vi "main.vi"() -> ()   [LabVIEW 2020]
doc: "Take photo if matching template."
uses:
  <vilib>/userDefined/High Color/IMAQdx.ctl
  <vilib>/Utility/error.llb/DialogType.ctl
  controls/Car Wash Data.ctl
  controls/Car Wash Entry Console.ctl
  controls/Car Wash Led.ctl
panel:
  in  "Stop program":bool
  in  "Tab Control":enum32{"Controls", "Statistics", "Admin Panel"}(tab)
  out "Reading ID":bool
  in  "Car ID":string
  in  "Car Position Slider":u16(slide) scale=0.0..4.0
  out "Under Body Wash":bool
  out "Bug Remover":bool
  out "Pre-Soak":bool
  out "High Pressure Wash":bool
  out "Low Pressure Wax":bool
  out "Spot Free Rinse":bool
  out "Tire Shine Foam":bool
  out "Air Dry":bool
  out "Vehicle Out Of Position":bool
  out "Elapsed Time":dbl format="%#_2g"
  out "Wash Entry":bool
  in  "Start":bool
  in  "Entry Console":T1
  out "Cleanest Car ID":string[](array[string])
  out "Histogram":cluster{"Options (1-8)":i32[], "Array":i64[]}(graph)
  out "Database":string[][](table)
  in  "Choose camera":T2="cam2"
  out "Current ID":string
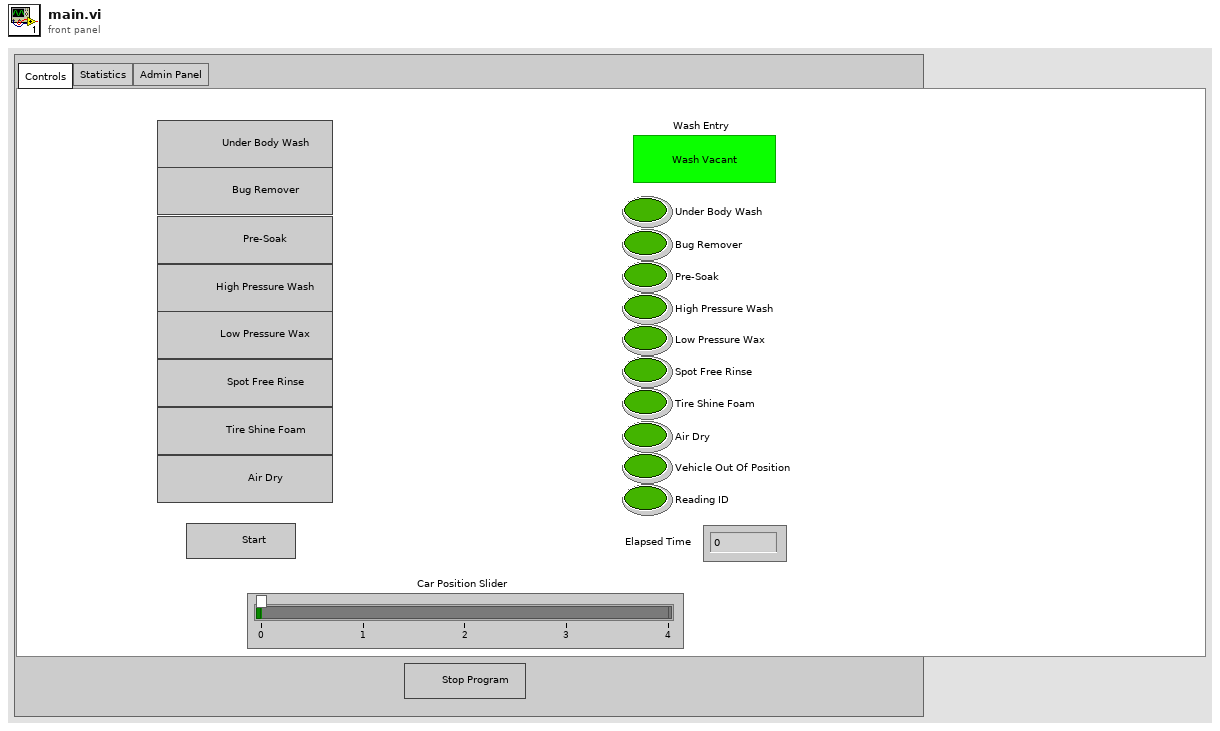
[diagram p1: front panel]
types:
  T1 = cluster{"Under Body Wash Button":bool, "Bug Remover Button":bool, "Pre-Soak Button":bool, "High Pressure Wash Button":bool, "Low Pressure Wax Button":bool, "Spot Free Rinse Button":bool, "Tire Shine Foam Button":bool, "Air Dry Button":bool}
  T2 = typedef "IMAQdx.ctl" = refnum<k21>
  T3 = enum32{"Invalid", "Standard", "Closed", "Hidden", "Minimized", "Maximized"}
  T4 = enum32{"invalid app kind", "Development System", "Run Time System", "Student Edition", "Embedded LabVIEW", "Evaluation", "Custom"}
  T5 = enum8{"Enabled", "Disabled", "Disabled and Grayed Out"}
  T6 = typedef "Car Wash Entry Console.ctl" = cluster{"Under Body Wash Button":bool, "Bug Remover Button":bool, "Pre-Soak Button":bool, "High Pressure Wash Button":bool, "Low Pressure Wax Button":bool, "Spot Free Rinse Button":bool, "Tire Shine Foam Button":bool, "Air Dry":bool}
  T7 = typedef "Car Wash Led.ctl" = cluster{"Under Body Wash":bool, "Bug Remover":bool, "Pre-Soak":bool, "High Pressure Wash":bool, "Low Pressure Wax":bool, "Spot Free Rinse":bool, "Tire Shine Foam":bool, "Air Dry":bool, "Vehicle out If Position":bool, "Wash Entry":bool, "Reading ID":bool}
  T8 = typedef "Car Wash Data.ctl" = cluster{"Entry Console":T6, "Car Wash Display":cluster{"Timer":dbl, "Reset Stoper":bool, "LED":T7, "Elapsed Time":dbl}, "Car Position Slider":u16, "Run Mode":bool}
  T9 = cluster{"Core":cluster{"Current VI Reference":refnum<vi>, "Close Panel on Exit?":bool}, "Car Wash Data":T8, "Car ID":string, "SQLite Connection":refnum<class "Connection.lvclass">}
  T10 = typedef "DialogType.ctl" = u16
  T11 = cluster{"Current VI Reference":refnum<vi>, "Close Panel on Exit?":bool}
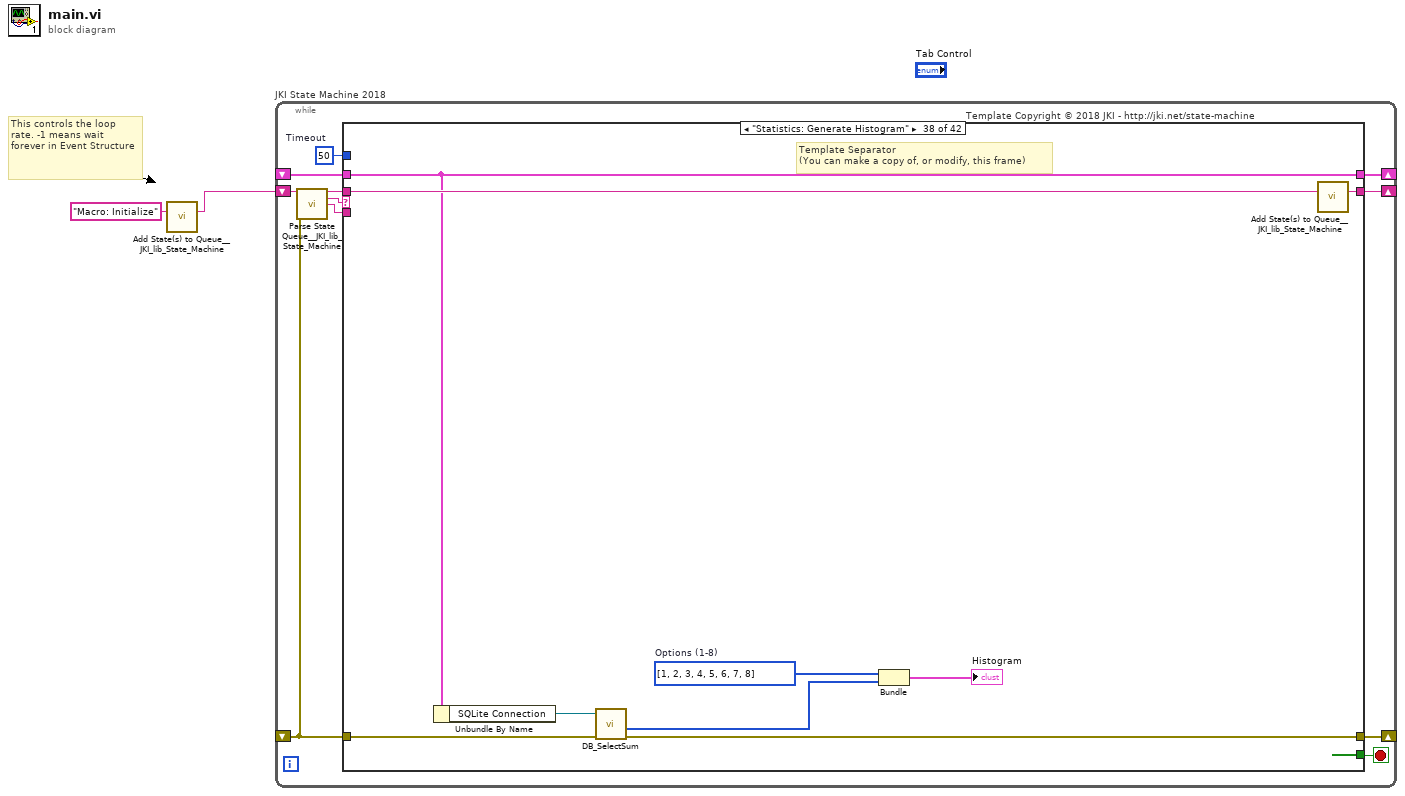
[diagram p0: block diagram]
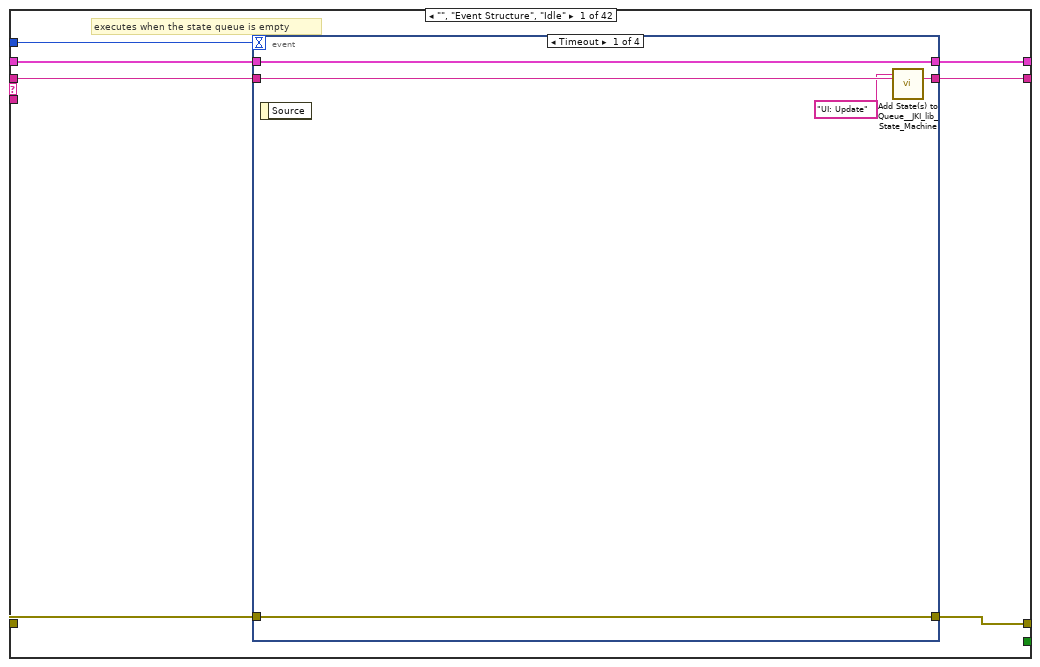
[diagram p2: hidden frame]
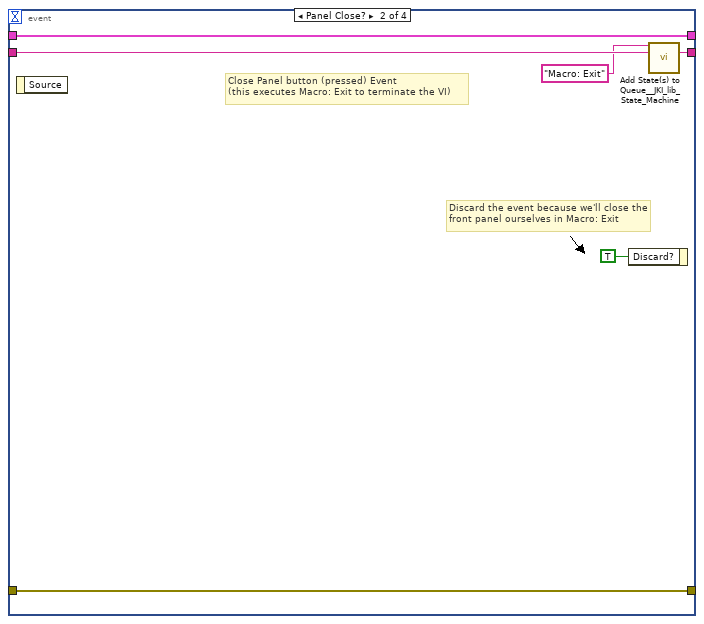
[diagram p3: hidden frame]
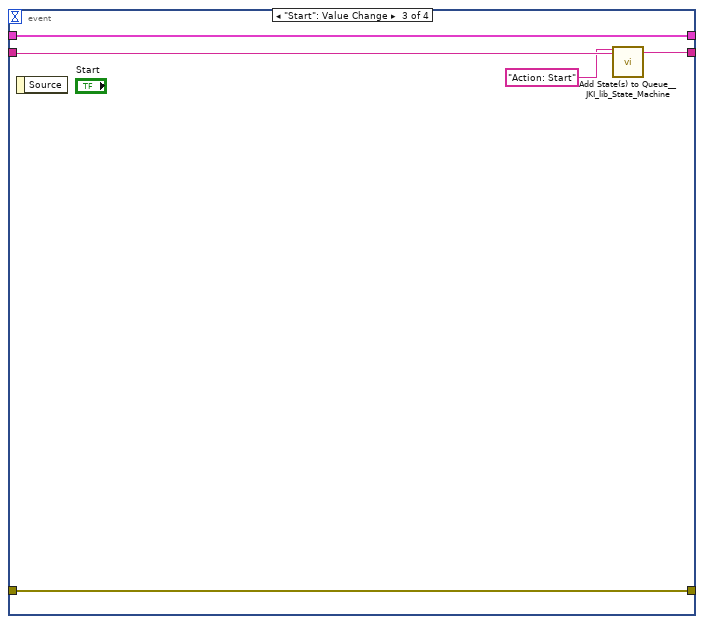
[diagram p4: hidden frame]
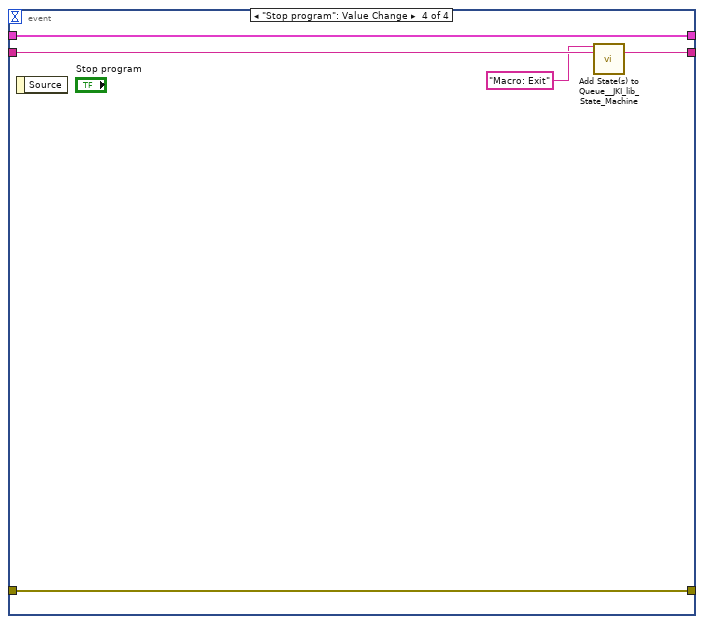
[diagram p5: hidden frame]
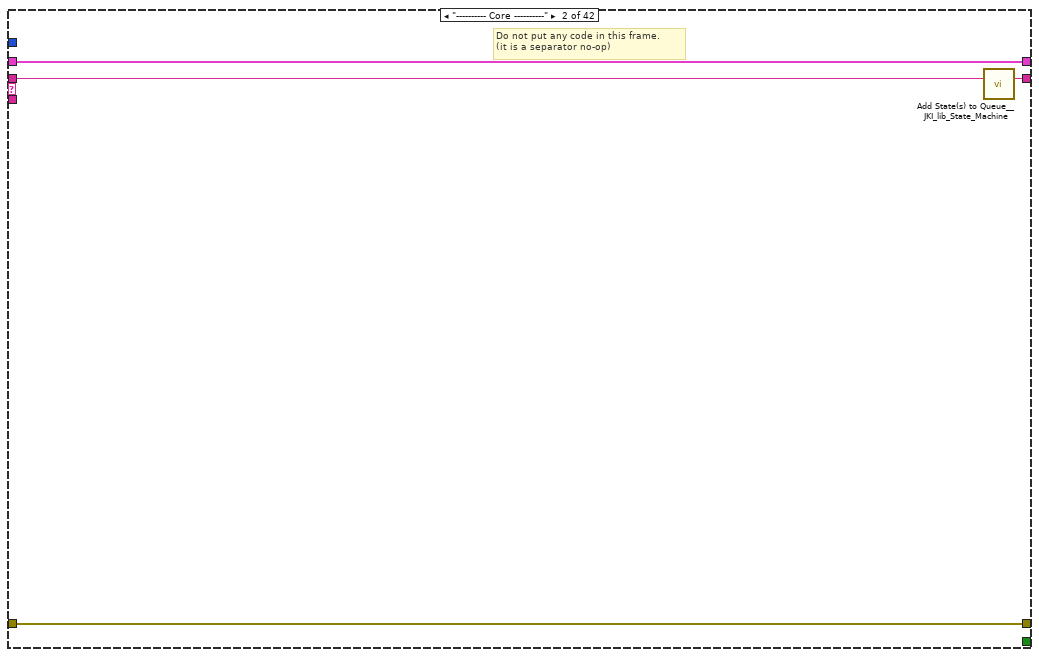
[diagram p6: hidden frame]
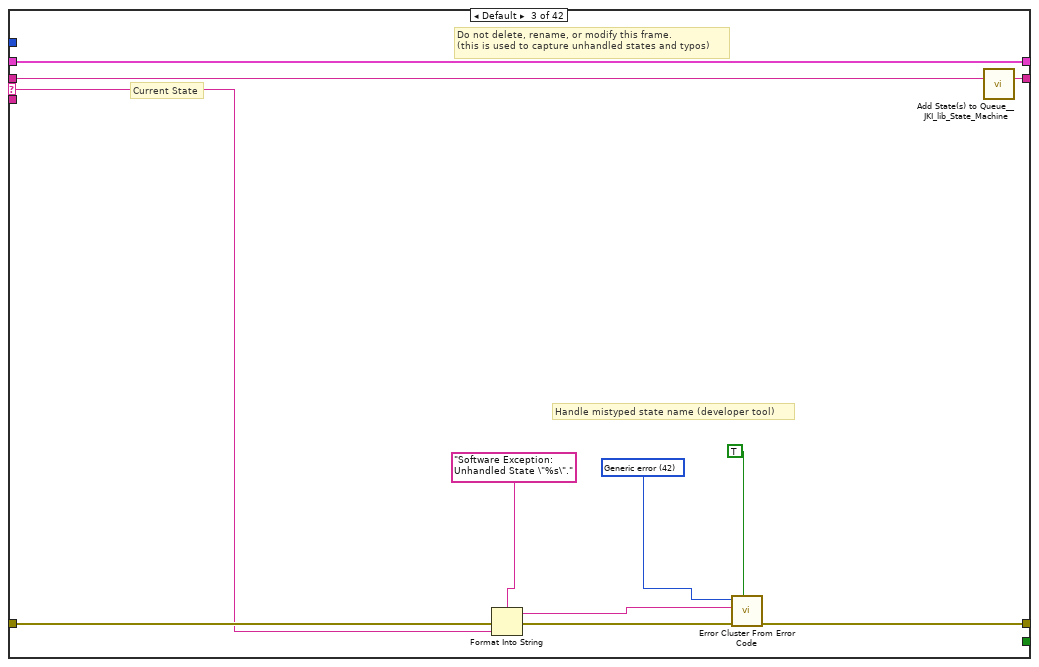
[diagram p7: hidden frame]
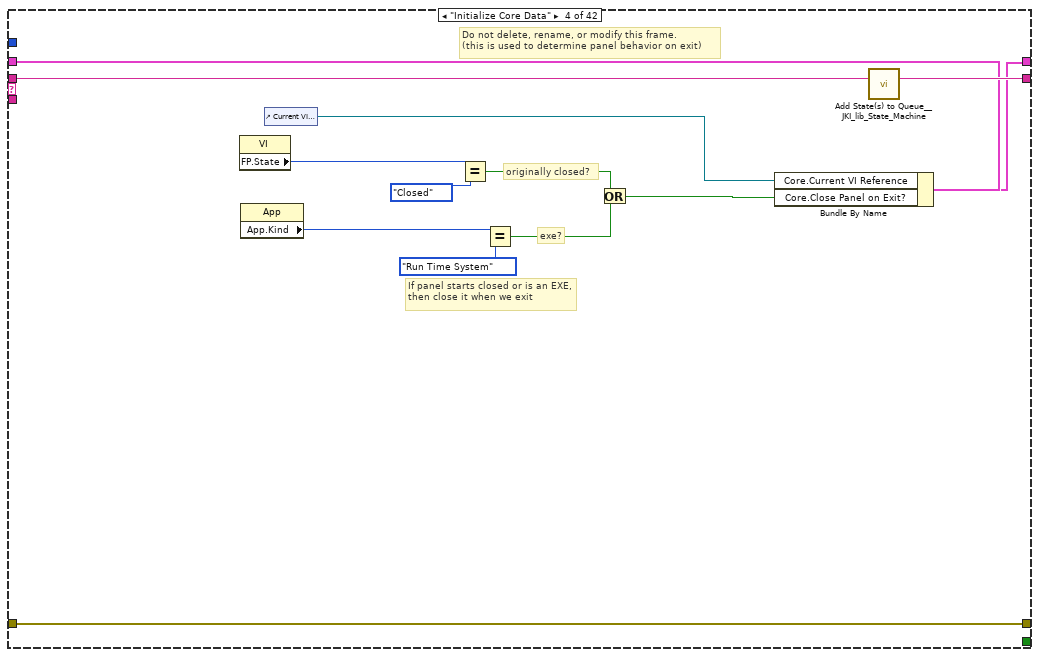
[diagram p8: hidden frame]
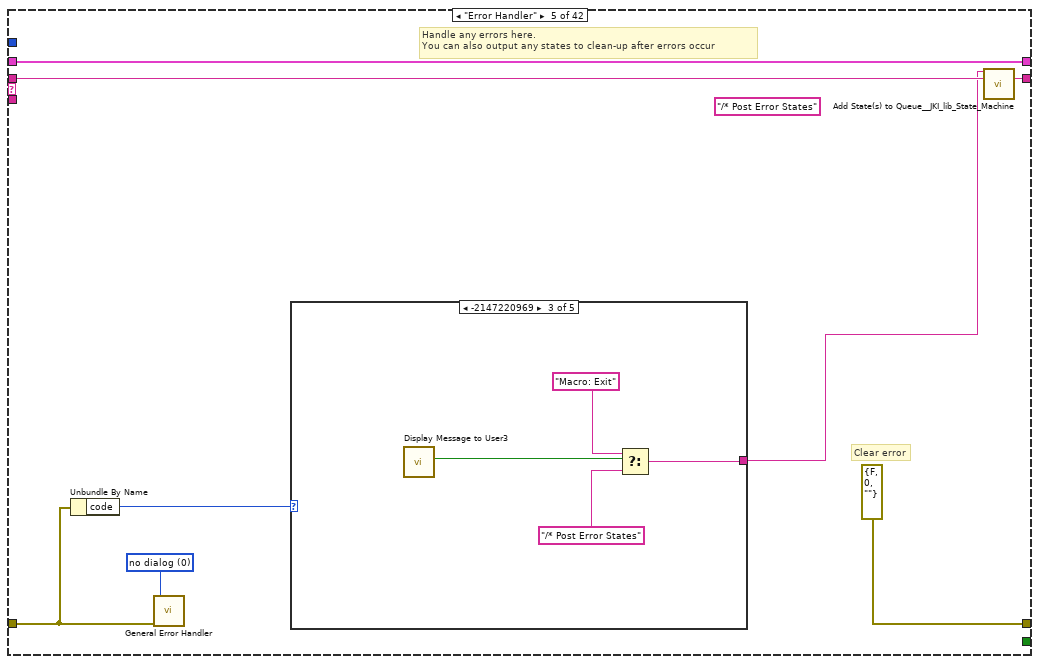
[diagram p9: hidden frame]
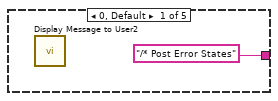
[diagram p10: hidden frame]
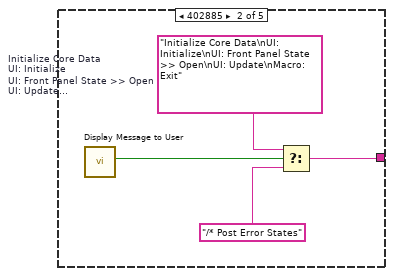
[diagram p11: hidden frame]
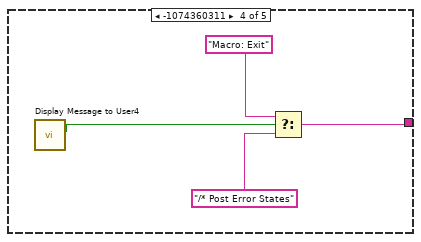
[diagram p12: hidden frame]
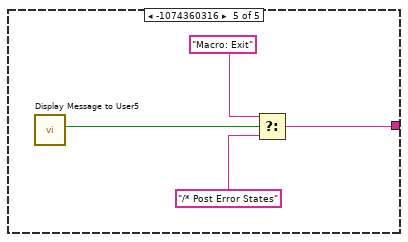
[diagram p13: hidden frame]
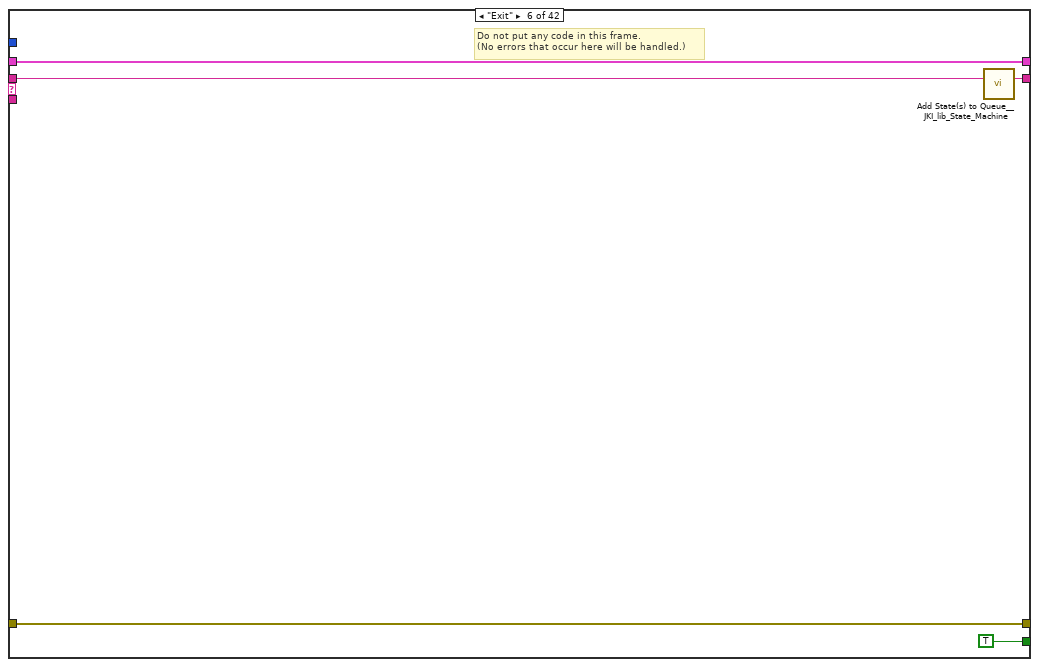
[diagram p14: hidden frame]
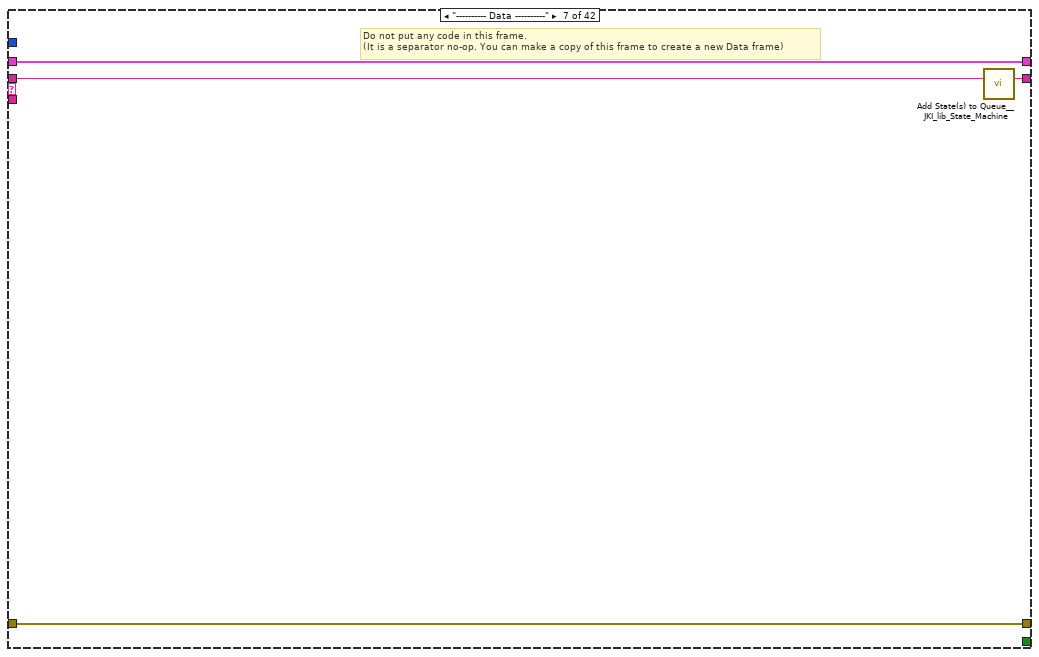
[diagram p15: hidden frame]
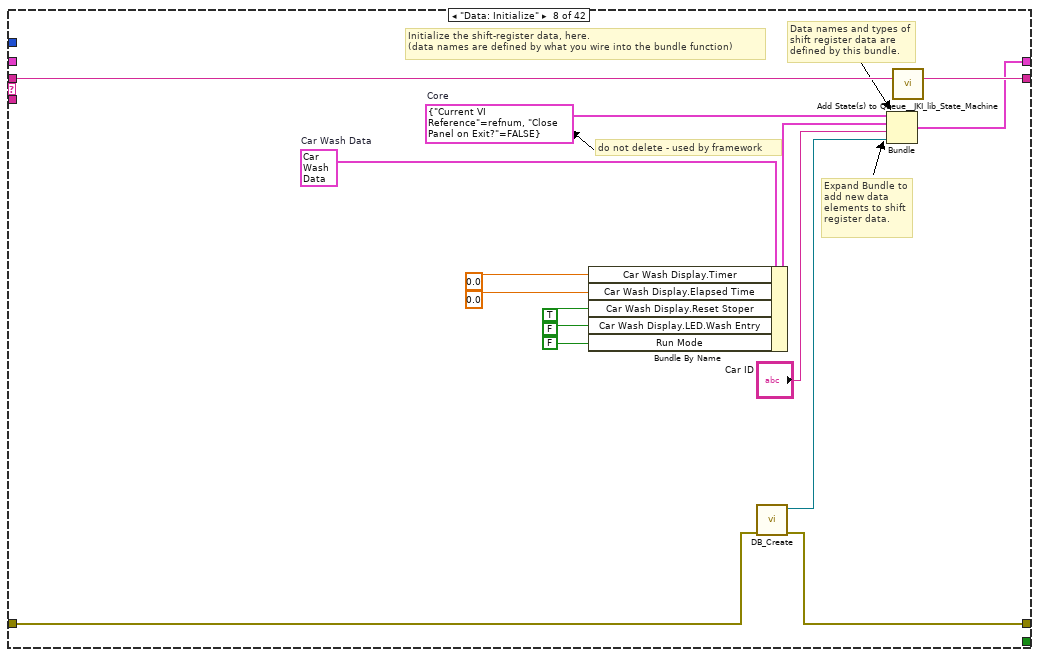
[diagram p16: hidden frame]
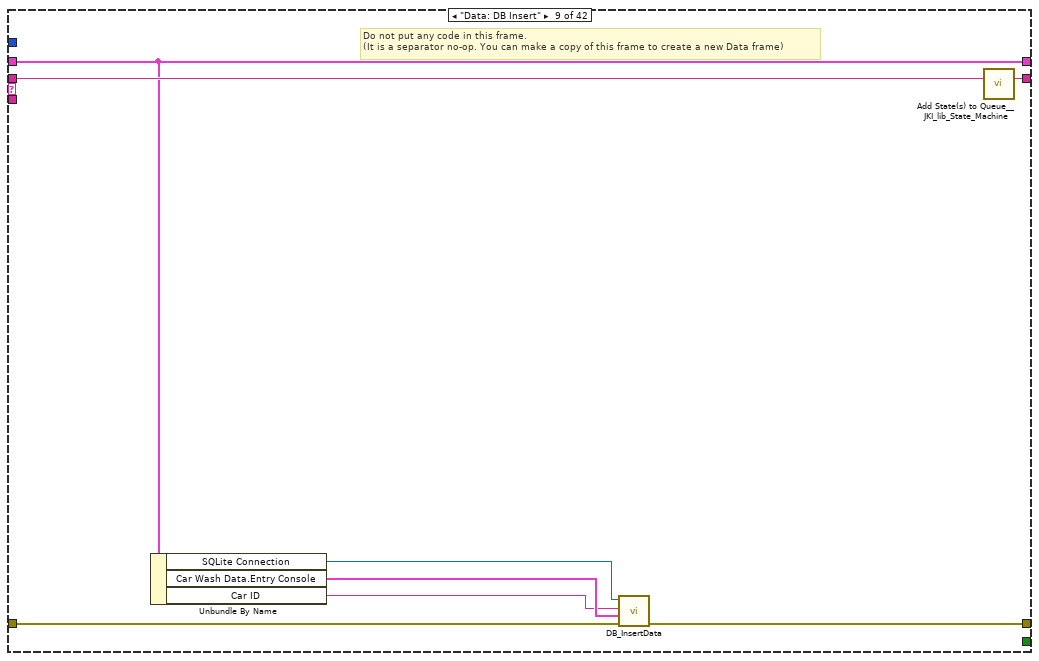
[diagram p17: hidden frame]
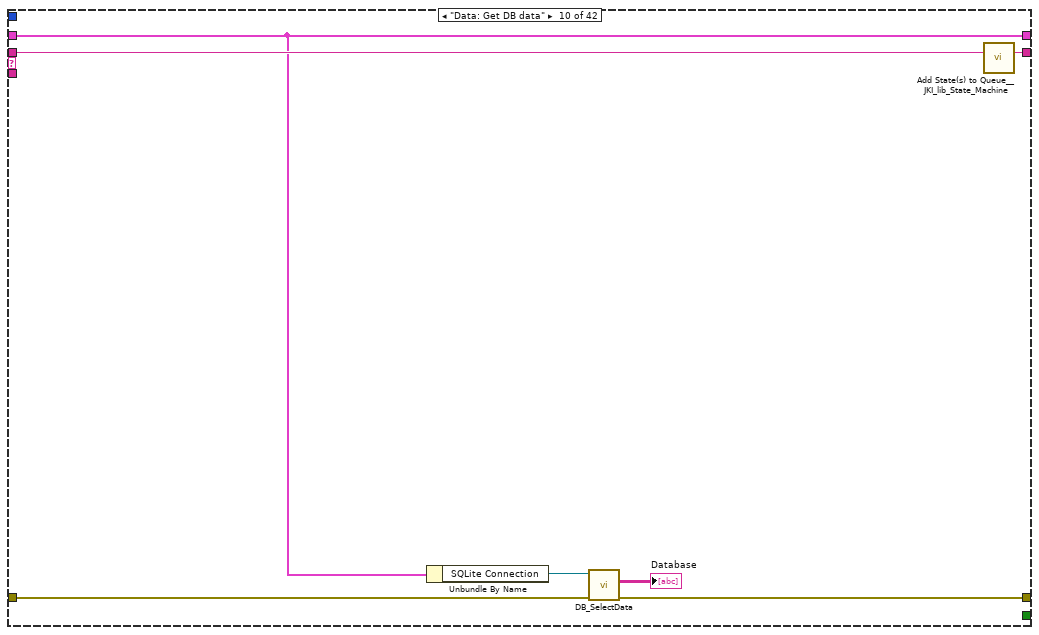
[diagram p18: hidden frame]
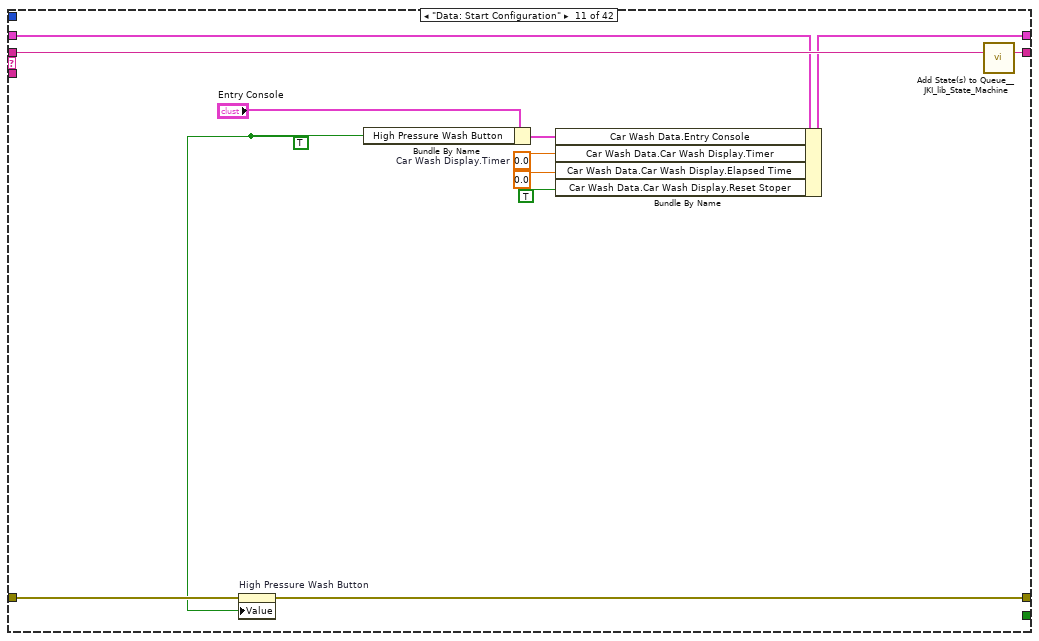
[diagram p19: hidden frame]
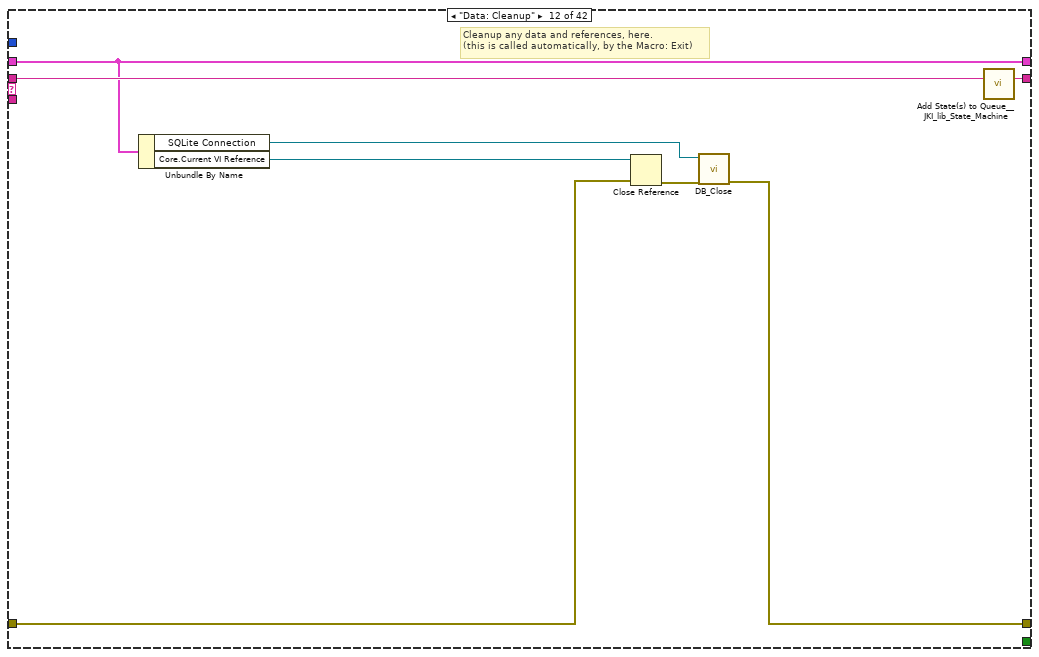
[diagram p20: hidden frame]
diagram:
  # "This controls the loop rate. -1 means wait forever in Event Structure"
  n1 = call <vilib>:"Add State(s) to Queue__JKI_lib_State_Machine.vi"("State(s) in (\"\")"="Macro: Initialize") -> ("States Out"=w2:string)  [unwired: 14 in]
  n2 = while "JKI State Machine 2018" {
    shift-right: [w6] -> _
    shift-left: _ -> [w5]
    shift-right: [w9] -> _
    shift-left: _ -> [w3]
    shift-right: [w8] -> _
    shift-left: w2 -> [w10]
    stop <- w7 stop-if-true
    w4 = 50  # Timeout
    # "Template Copyright © 2018 JKI - http://jki.net/state-machine"
    n3 = call <vilib>:"Parse State Queue__JKI_lib_State_Machine.vi"("State Queue"=w10, "Error In (no error)"=w3) -> ("Remaining States"=w12:string, "Current State"=w13:string, "Arguments"=w11:string)  [unwired: 11 in]
    n4 = case shown="\"Statistics: Generate Histogram\"" w13 {
      selector: w13 -> [_ _ w46 _ _ _ _ _ _ _ _ _ _ _ _ _ _ _ _ _ _ _ _ _ _ _ _ _ _ _ _ _ _ _ _ _ _ _ _ _ _ _]
      tunnel: w12 -> [w20 w45 w50 w69 w77 w99 w103 w118 w123 w133 w145 w153 w157 w171 w177 w188 w269 w276 w281 w286 w291 w296 w306 w310 w315 w329 w341 w362 w383 w404 w425 w446 w467 w488 w510 w541 w545 w554 w561 w565 w575 w584]
      tunnel: w11 -> [_ _ _ _ _ _ _ _ _ _ _ _ _ _ w172 w183 _ _ _ _ _ _ _ _ _ _ _ _ _ _ _ _ _ _ _ _ _ _ _ _ _ _]
      tunnel: w5 -> [w18 w42 w48 w58 w74 w97 w100 _ w122 w131 w139 w151 w154 w169 w175 w182 w256 w273 w278 w283 w288 w293 w299 w307 w312 w326 w348 w369 w390 w411 w432 w453 w474 w495 w503 w535 w542 w552 w559 w562 w571 w578]
      tunnel: [w17 w43 w52 w67 errorcluster {"status"=FALSE, "code"=0, "source"=""} ("error out") w96 w101 w108 w124 w129 w135 w146 w155 w161 w173 w185 w251 w274 w279 w284 w289 w294 w304 w308 w311 w322 w344 w365 w386 w407 w428 w449 w470 w491 w505 w538 w543 w551 w557 w563 w568 w581] -> w9
      tunnel: w3 -> [w16 w43 w51 w67 w73 w96 w101 w107 w121 w130 w136 w148 w155 w158 w174 w186 w250 w274 w279 w284 w289 w294 w304 w308 w311 w318 w343 w364 w385 w406 w427 w448 w469 w490 w506 w530 w543 w550 w558 w563 w567 w582]
      tunnel: [w19 w44 w49 w68 w76 w98 w102 w117 w126 w132 w144 w152 w156 w170 w176 w187 w268 w275 w280 w285 w290 w295 w305 w309 w314 w328 w350 w371 w392 w413 w434 w455 w476 w497 w509 w540 w544 w553 w560 w564 w574 w583] -> w8
      tunnel: [_ _ _ _ _ TRUE _ _ _ _ _ _ _ _ _ _ _ _ _ _ _ _ _ _ _ _ _ _ _ _ _ _ _ _ _ _ _ _ _ _ _ _] -> w7
      tunnel: [w14 w42 w48 w57 w74 w97 w100 w114 w122 w131 w140 w151 w154 w169 w175 w182 w257 w273 w278 w283 w288 w293 w299 w307 w312 w327 w349 w370 w391 w412 w433 w454 w475 w496 w502 w536 w542 w552 w559 w562 w571 w579] -> w6
      tunnel: w4 -> [w15 _ _ _ _ _ _ _ _ _ _ _ _ _ _ _ _ _ _ _ _ _ _ _ _ _ _ _ _ _ _ _ _ _ _ _ _ _ _ _ _ _]
      frame "", "Event Structure", "Idle" {
        # "executes when the state queue is empty"
        n5 = event shown="[0] Timeout" {
          selector: _ -> [_ _ _ _]
          dyn-events: _ -> [_ _ _ _]
          timeout: w15 -> [_ _ _ _]
          tunnel: w20 -> [w25 w31 w33 w41]
          tunnel: [w24 w30 w36 w40] -> w19
          tunnel: w18 -> [w22 w28 w35 w38]
          tunnel: [w23 w29 w34 w37] -> w17
          tunnel: w16 -> [w23 w29 w34 w37]
          tunnel: [w22 w28 w35 w38] -> w14
          event Timeout {
            n6 = event-data() -> ()  [unwired: 1 in, 1 out]
            n7 = call <vilib>:"Add State(s) to Queue__JKI_lib_State_Machine.vi"("State(s) in Front (\"\")"="UI: Update" ("State(s) at Back (\"\")"), "State(s) in (\"\")"=w25) -> ("States Out"=w24:string)  [unwired: 13 in]
          }
          event Panel Close? {
            # "Discard the event because we'll close the front panel ourselves in Macro: Exit"
            # "Close Panel button (pressed) Event\n(this executes Macro: Exit to terminate the VI)"
            n8 = event-data() -> ()  [unwired: 1 in, 1 out]
            n9 = event-data("Discard?"=TRUE) -> ()  [unwired: 1 in, 1 out]
            n10 = call <vilib>:"Add State(s) to Queue__JKI_lib_State_Machine.vi"("State(s) in Front (\"\")"="Macro: Exit", "State(s) in (\"\")"=w31) -> ("States Out"=w30:string)  [unwired: 13 in]
          }
          event "Start": Value Change {
            n11 = event-data() -> ()  [unwired: 1 in, 1 out]
            n12 = call <vilib>:"Add State(s) to Queue__JKI_lib_State_Machine.vi"("State(s) in Front (\"\")"="Action: Start", "State(s) in (\"\")"=w33) -> ("States Out"=w36:string)  [unwired: 13 in]
          }
          event "Stop program": Value Change {
            n13 = event-data() -> ()  [unwired: 1 in, 1 out]
            n14 = call <vilib>:"Add State(s) to Queue__JKI_lib_State_Machine.vi"("State(s) in Front (\"\")"="Macro: Exit", "State(s) in (\"\")"=w41) -> ("States Out"=w40:string)  [unwired: 13 in]
          }
        }
      }
      frame "---------- Core ----------" {
        # "Do not put any code in this frame.\n(it is a separator no-op)"
        n15 = call <vilib>:"Add State(s) to Queue__JKI_lib_State_Machine.vi"("State(s) in (\"\")"=w45) -> ("States Out"=w44:string)  [unwired: 14 in]
      }
      frame Default {
        w55 = 42 items=["No error", "Argument error", "Memory is full", "Out of zone", "End of file", "File already open", "Generic file I/O error", "File not found", "File permission error", "Disk is full", "Duplicate path", "Too many files open", "System feature not enabled", "Resource file not found", "Cannot add resource", "Resource not found", "Image not found", "Image memory error", "Pen does not exist", "Config type invalid", "Config token not found", "Config parse error", "Config memory error", "Bad external code format", "Bad external code offset", "External code not present", "Null window", "Destroy window error", "Null menu", "Print aborted", "Bad print record", "Print driver error", "Windows error during printing", "Memory error during printing", "Print dialog error", "Generic print error", "Invalid device refnum", "Device not found", "Device parameter error", "Device unit error", "Cannot open device", "Device call aborted", "Generic error", "Cancelled by user", "Object ID too low", "Object ID too high", "Object not in heap", "Unknown heap", "Unknown object (invalid DefProc)", "Unknown object (DefProc not in table)", "Message out of range", "Invalid (null) method", "Unknown message", "Manager call not supported", "Bad address", "Network operation in progress", "Network operation timed out", "Connection is busy", "Network attribute not supported", "Network error", "Address in use", "System out of memory", "Connection aborted", "Connection refused", "Not connected", "Already connected", "Connection closed", "Initialization error (interapplication manager)", "Bad occurrence", "Wait on unbound occurrence handler", "Occurrence queue overflow", "Datalog type conflict", "Unused", "Unrecognized type (interapplication manager)", "Memory corrupt", "Failed to make temporary DLL", "Old CIN version", "Drag socket not found", "Failed to load drop-object", "Failed to register OLE object", "Failed to release OLE object", "Format specifier type mismatch", "Unknown format specifier", "Too few format specifiers", "Too many format specifiers", "Scan failed", "Newer CIN version", "Error converting to variant", "Runtime menu error", "Password tampered", "Variant attribute not found", "Incompatible variant data type", "Event data is not available", "Event Store is not present", "Occurrence is not found", "Event Queue is not created", "Event info is not available", "Refnum passed is NULL", "Error retrieving Class GUID", "Error retrieving CoClass GUID", "Error retrieving TypeLib GUID.", "Bad built application magic bytes.", "Specific driver is different from the specific driver associated with the Logical Name.", "There is no session opened to the class driver.", "Max Error", "MAX - Error with config objects", "MAX - Error loading configuration", "MAX - Group not supported"]
        # "Current State"
        # "Do not delete, rename, or modify this frame.\n(this is used to capture unhandled states and typos)"
        # "Handle mistyped state name (developer tool)"
        n16 = Format Into String(format string="Software Exception: Unhandled State \"%s\"." ("message"), error in=w51, w46) -> (resulting string=w54:string, error out=w53:errorcluster)  [unwired: 1 in]
        n17 = call <vilib>:"Error Cluster From Error Code.vi"("show call chain? (False)"=TRUE, "error in (no error)"=w53, "error message (\"\")"=w54, "error code (0)"=w55) -> ("error out"=w52:errorcluster)  [unwired: 5 in]
        n18 = call <vilib>:"Add State(s) to Queue__JKI_lib_State_Machine.vi"("State(s) in (\"\")"=w50) -> ("States Out"=w49:string)  [unwired: 14 in]
      }
      frame "Initialize Core Data" {
        # "Do not delete, rename, or modify this frame.\n(this is used to determine panel behavior on exit)"
        # "originally closed?"
        # "exe?"
        # "If panel starts closed or is an EXE, then close it when we exit"
        n19 = property class="VI"() -> ("FP.State"=w61:T3)  [unwired: 2 in, 2 out]
        n20 = property class="App"() -> ("App.Kind"=w66:T4)  [unwired: 2 in, 2 out]
        n21 = control-ref of="Current VI Reference"() -> (w62:refnum<vi>)
        n22 = Equal?(x=w61, y=T3."Closed" ("Front Panel Window:State")) -> (x = y?=w59:bool)
        n23 = Equal?(x=w66, y=T4."Run Time System" ("Application:Kind")) -> (x = y?=w64:bool)
        n24 = Or(x=w59, y=w64) -> (x .or. y?=w63:bool)
        n25 = Bundle By Name(cluster=w58, "Core.Current VI Reference"=w62, "Core.Close Panel on Exit?"=w63) -> (w57:T9)
        n26 = call <vilib>:"Add State(s) to Queue__JKI_lib_State_Machine.vi"("State(s) in (\"\")"=w69) -> ("States Out"=w68:string)  [unwired: 14 in]
      }
      frame "Error Handler" {
        w71 = T10 0 items=["no dialog", "OK message", "continue or stop message", "OK message + warnings", "continue/stop + warnings"] ("type of dialog (OK msg:1)")
        (unwired) "/* Post Error States"
        # "Handle any errors here.\nYou can also output any states to clean-up after errors occur"
        # "Clear error"
        n27 = Unbundle By Name(w73) -> ("code"=w72:i32)
        n28 = call <vilib>:"General Error Handler.vi"("type of dialog (OK msg:1)"=w71, "error in (no error)"=w73) -> ()  [unwired: 9 in, 5 out]
        n29 = case shown="-2147220969" w72 {
          tunnel: ["/* Post Error States" w79 w84 w88 w91] -> w70
          frame 0, Default {
            n30 = call "Display Message to User2"() -> ()  [unwired: 10 in, 2 out]
          }
          frame 402885 {
            w80 = "Initialize Core Data\nUI: Initialize\nUI: Front Panel State >> Open\nUI: Update\nMacro: Exit"  # Initialize Core Data UI: Initialize UI: Front Panel State >> Open UI: Update Macro: Exit
            n31 = call "Display Message to User"() -> ("STOP"=w81:bool)  [unwired: 10 in, 1 out]
            n32 = Select(t=w80, s=w81, f="/* Post Error States") -> (s? t:f=w79:string)
          }
          frame -2147220969 {
            n33 = call "Display Message to User3"() -> ("STOP"=w83:bool)  [unwired: 10 in, 1 out]
            n34 = Select(t="Macro: Exit", s=w83, f="/* Post Error States") -> (s? t:f=w84:string)
          }
          frame -1074360311 {
            n35 = call "Display Message to User4"() -> ("STOP"=w87:bool)  [unwired: 10 in, 1 out]
            n36 = Select(t="Macro: Exit", s=w87, f="/* Post Error States") -> (s? t:f=w88:string)
          }
          frame -1074360316 {
            n37 = call "Display Message to User5"() -> ("STOP"=w92:bool)  [unwired: 10 in, 1 out]
            n38 = Select(t="Macro: Exit", s=w92, f="/* Post Error States") -> (s? t:f=w91:string)
          }
        }
        n39 = call <vilib>:"Add State(s) to Queue__JKI_lib_State_Machine.vi"("State(s) in Front (\"\")"=w70, "State(s) in (\"\")"=w77) -> ("States Out"=w76:string)  [unwired: 13 in]
      }
      frame "Exit" {
        # "Do not put any code in this frame.\n(No errors that occur here will be handled.)"
        n40 = call <vilib>:"Add State(s) to Queue__JKI_lib_State_Machine.vi"("State(s) in (\"\")"=w99) -> ("States Out"=w98:string)  [unwired: 14 in]
      }
      frame "---------- Data ----------" {
        # "Do not put any code in this frame.\n(It is a separator no-op. You can make a copy of this frame to create a new Data frame)"
        n41 = call <vilib>:"Add State(s) to Queue__JKI_lib_State_Machine.vi"("State(s) in (\"\")"=w103) -> ("States Out"=w102:string)  [unwired: 14 in]
      }
      frame "Data: Initialize" {
        w116 = T8 {"Entry Console"={"Under Body Wash Button"=FALSE, "Bug Remover Button"=FALSE, "Pre-Soak Button"=FALSE, "High Pressure Wash Button"=FALSE, "Low Pressure Wax Button"=FALSE, "Spot Free Rinse Button"=FALSE, "Tire Shine Foam Button"=FALSE, "Air Dry"=FALSE}, "Car Wash Display"={"Timer"=0.0, "Reset Stoper"=FALSE, "LED"={"Under Body Wash"=FALSE, "Bug Remover"=FALSE, "Pre-Soak"=FALSE, "High Pressure Wash"=FALSE, "Low Pressure Wax"=FALSE, "Spot Free Rinse"=FALSE, "Tire Shine Foam"=FALSE, "Air Dry"=FALSE, "Vehicle out If Position"=FALSE, "Wash Entry"=FALSE, "Reading ID"=FALSE}, "Elapsed Time"=0.0}, "Car Position Slider"=0, "Run Mode"=FALSE}  # Car Wash Data
        w109 = T11 {"Current VI Reference"=refnum, "Close Panel on Exit?"=FALSE}  # Core
        # "do not delete - used by framework"
        # "Expand Bundle to add new data elements to shift register data."
        # "Data names and types of shift register data are defined by this bundle."
        # "Initialize the shift-register data, here.\n(data names are defined by what you wire into the bundle function)"
        n42 = Bundle By Name(cluster=w116, "Car Wash Display.Timer"=0.0, "Car Wash Display.Elapsed Time"=0.0, "Car Wash Display.Reset Stoper"=TRUE, "Car Wash Display.LED.Wash Entry"=FALSE, "Run Mode"=FALSE) -> (w115:T8)
        n43 = call "DB_Create.vi"("error in"=w107) -> ("error out"=w108:errorcluster, "SQLite Connection"=w106:refnum<class "Connection.lvclass">)  [unwired: 9 in]
        n44 = Bundle("Core"=w109, "Car Wash Data"=w115, "Car ID"="Car ID", "SQLite Connection"=w106) -> (w114:T9)  [unwired: 1 in]
        n45 = call <vilib>:"Add State(s) to Queue__JKI_lib_State_Machine.vi"("State(s) in (\"\")"=w118) -> ("States Out"=w117:string)  [unwired: 14 in]
      }
      frame "Data: DB Insert" {
        # "Do not put any code in this frame.\n(It is a separator no-op. You can make a copy of this frame to create a new Data frame)"
        n46 = Unbundle By Name(w122) -> ("SQLite Connection"=w125:refnum<class "Connection.lvclass">, "Car Wash Data.Entry Console"=w120:T6, "Car ID"=w119:string)
        n47 = call "DB_InsertData.vi"("error in (no error)"=w121, "Entry Console"=w120, "ID"=w119, "SQLite Connection in"=w125) -> ("error out"=w124:errorcluster)  [unwired: 6 in, 1 out]
        n48 = call <vilib>:"Add State(s) to Queue__JKI_lib_State_Machine.vi"("State(s) in (\"\")"=w123) -> ("States Out"=w126:string)  [unwired: 14 in]
      }
      frame "Data: Get DB data" {
        n49 = Unbundle By Name(w131) -> ("SQLite Connection"=w128:refnum<class "Connection.lvclass">)
        n50 = call "DB_SelectData.vi"("error in (no error)"=w130, "SQLite Connection in"=w128) -> ("error out"=w129:errorcluster, "Data"=→"Database":string[][])  [unwired: 7 in, 1 out]
        n51 = call <vilib>:"Add State(s) to Queue__JKI_lib_State_Machine.vi"("State(s) in (\"\")"=w133) -> ("States Out"=w132:string)  [unwired: 14 in]
      }
      frame "Data: Start Configuration" {
        w134 = TRUE ("High Pressure Wash Button")
        w143 = 0.0  # Car Wash Display.Timer
        n52 = property on="High Pressure Wash Button" class="Bool (strict)"(error in=w136, "Value"=w134) -> (error out=w135:errorcluster)  [unwired: 1 in, 1 out]
        n53 = Bundle By Name(cluster="Entry Console", "High Pressure Wash Button"=w134) -> (w138:T1)
        n54 = Bundle By Name(cluster=w139, "Car Wash Data.Entry Console"=w138, "Car Wash Data.Car Wash Display.Timer"=w143, "Car Wash Data.Car Wash Display.Elapsed Time"=0.0 ("Car Wash Display.Elapsed Time"), "Car Wash Data.Car Wash Display.Reset Stoper"=TRUE ("Car Wash Display.Reset Stoper")) -> (w140:T9)
        n55 = call <vilib>:"Add State(s) to Queue__JKI_lib_State_Machine.vi"("State(s) in (\"\")"=w145) -> ("States Out"=w144:string)  [unwired: 14 in]
      }
      frame "Data: Cleanup" {
        # "Cleanup any data and references, here.\n(this is called automatically, by the Macro: Exit)"
        n56 = Unbundle By Name(w151) -> ("SQLite Connection"=w149:refnum<class "Connection.lvclass">, "Core.Current VI Reference"=w150:refnum<vi>)
        n57 = Close Reference(reference=w150, error in (no error)=w148) -> (error out=w147:errorcluster)
        n58 = call "DB_Close.vi"("error in (no error)"=w147, "SQLite Connection in"=w149) -> ("error out"=w146:errorcluster)  [unwired: 9 in]
        n59 = call <vilib>:"Add State(s) to Queue__JKI_lib_State_Machine.vi"("State(s) in (\"\")"=w153) -> ("States Out"=w152:string)  [unwired: 14 in]
      }
      frame "---------- UI ----------" {
        # "Do not put any code in this frame.\n(It is a separator no-op. You can make a copy of this frame to create a new UI frame)"
        n60 = call <vilib>:"Add State(s) to Queue__JKI_lib_State_Machine.vi"("State(s) in (\"\")"=w157) -> ("States Out"=w156:string)  [unwired: 14 in]
      }
      frame "UI: Initialize" {
        w162 = u16 0 items=["Entry", "Station 1", "Station 2", "Station 3", "Exit"] ("Car Position Slider")
        # "Initialize the User Interface, here.\n(this is called automatically, by the Macro: Init)"
        n61 = property on="Current ID" class="Str"(error in=w158, "Value"="") -> (error out=w159:errorcluster)  [unwired: 1 in, 1 out]
        n62 = property on="Entry Console" class="Clust (strict)"(error in=w159, "DisabledEnum"=T5."Enabled" ("Disabled")) -> (error out=w168:errorcluster)  [unwired: 1 in, 1 out]
        n63 = property on="Entry Console" class="Clust (strict)"(error in=w168, "Value"=T6 {"Under Body Wash Button"=FALSE, "Bug Remover Button"=FALSE, "Pre-Soak Button"=FALSE, "High Pressure Wash Button"=FALSE, "Low Pressure Wax Button"=FALSE, "Spot Free Rinse Button"=FALSE, "Tire Shine Foam Button"=FALSE, "Air Dry"=FALSE} ("Entry Console")) -> (error out=w167:errorcluster)  [unwired: 1 in, 1 out]
        n64 = property on="Car Position Slider" class="Slide (strict)"(error in=w167, "Value"=w162) -> (error out=w166:errorcluster)  [unwired: 1 in, 1 out]
        n65 = property on="Car Position Slider" class="Slide (strict)"(error in=w166, "DisabledEnum"=T5."Disabled" ("Disabled")) -> (error out=w161:errorcluster)  [unwired: 1 in, 1 out]
        n66 = call <vilib>:"Add State(s) to Queue__JKI_lib_State_Machine.vi"("State(s) in (\"\")"=w171) -> ("States Out"=w170:string)  [unwired: 14 in]
      }
      frame "UI: Cursor Set" {
        # "Argument"
        # "Set and Unset Cursor Busy.\n(Usage: \"UI: Cursor Set >> Busy|Idle\")"
        n67 = case shown="\"Idle\", Default" w172 {
          tunnel: w174 -> [w179 w181]
          tunnel: [w178 w180] -> w173
          frame "Idle", Default {
            n68 = call <vilib>:"Unset Busy.vi"("error in (no error)"=w179) -> ("error out"=w178:errorcluster)  [unwired: 10 in]
          }
          frame "Busy" {
            n69 = call <vilib>:"Set Busy.vi"("error in (no error)"=w181) -> ("error out"=w180:errorcluster)  [unwired: 9 in, 1 out]
          }
        }
        n70 = call <vilib>:"Add State(s) to Queue__JKI_lib_State_Machine.vi"("State(s) in (\"\")"=w177) -> ("States Out"=w176:string)  [unwired: 14 in]
      }
      frame "UI: Front Panel State" {
        # "Argument"
        # "Set Front Panel Open or Closed\n(Usage: \"UI: Front Panel State >> Open|Close\")"
        n71 = Unbundle By Name(w182) -> ("Core.Current VI Reference"=w184:refnum<vi>)
        n72 = case shown="\"Open\", \"Standard\", Default" w183 {
          tunnel: w186 -> [w194 w207 w218 w230 w242]
          tunnel: [w195 w208 w219 w231 w243] -> w185
          tunnel: w184 -> [_ _ _ _ _]
          frame "Open", "Standard", Default {
            w189 = T3."Standard" ("State")
            n73 = property class="VI"(error in=w194) -> (reference out=w192:refnum<vi>, error out=w193:errorcluster, "FP.State"=w191:T3)  [unwired: 1 in]
            n74 = Not Equal?(x=w191, y=w189) -> (x != y?=w190:bool)
            n75 = case shown="False" w190 {
              tunnel: [w199 w201] -> w195
              tunnel: w193 -> [w198 w201]
              tunnel: w192 -> [w197 _]
              tunnel: w189 -> [w196 _]
              frame True {
                n76 = invoke class="VI" method="FP.Open"(reference=w197, error in=w198, "Activate"=TRUE, "State"=w196) -> (error out=w199:errorcluster)  [unwired: 1 in, 4 out]
              }
              frame False {
              }
            }
          }
          frame "Close", "Closed" {
            n77 = property class="VI"(error in=w207) -> (reference out=w205:refnum<vi>, error out=w206:errorcluster, "FP.State"=w203:T3)  [unwired: 1 in]
            n78 = Not Equal?(x=w203, y=T3."Closed" ("Front Panel Window:State")) -> (x != y?=w202:bool)
            n79 = case shown="True" w202 {
              tunnel: [w209 w212] -> w208
              tunnel: w206 -> [w209 w211]
              tunnel: w205 -> [_ w210]
              frame False {
              }
              frame True {
                n80 = invoke class="VI" method="FP.Close"(reference=w210, error in=w211) -> (error out=w212:errorcluster)  [unwired: 1 in, 2 out]
              }
            }
          }
          frame "Hidden", "Hide" {
            w213 = T3."Hidden" ("State")
            n81 = property class="VI"(error in=w218) -> (reference out=w216:refnum<vi>, error out=w217:errorcluster, "FP.State"=w215:T3)  [unwired: 1 in]
            n82 = Not Equal?(x=w215, y=w213) -> (x != y?=w214:bool)
            n83 = case shown="True" w214 {
              tunnel: [w223 w224] -> w219
              tunnel: w217 -> [w222 w224]
              tunnel: w216 -> [w221 _]
              tunnel: w213 -> [w220 _]
              frame True {
                n84 = invoke class="VI" method="FP.Open"(reference=w221, error in=w222, "State"=w220) -> (error out=w223:errorcluster)  [unwired: 2 in, 4 out]
              }
              frame False {
              }
            }
          }
          frame "Minimize", "Minimized" {
            w225 = T3."Minimized" ("State")
            n85 = property class="VI"(error in=w230) -> (reference out=w228:refnum<vi>, error out=w229:errorcluster, "FP.State"=w227:T3)  [unwired: 1 in]
            n86 = Not Equal?(x=w227, y=w225) -> (x != y?=w226:bool)
            n87 = case shown="True" w226 {
              tunnel: [w235 w236] -> w231
              tunnel: w229 -> [w234 w236]
              tunnel: w228 -> [w233 _]
              tunnel: w225 -> [w232 _]
              frame True {
                n88 = invoke class="VI" method="FP.Open"(reference=w233, error in=w234, "State"=w232) -> (error out=w235:errorcluster)  [unwired: 2 in, 4 out]
              }
              frame False {
              }
            }
          }
          frame "Maximize", "Maximized" {
            w237 = T3."Maximized" ("State")
            n89 = property class="VI"(error in=w242) -> (reference out=w240:refnum<vi>, error out=w241:errorcluster, "FP.State"=w239:T3)  [unwired: 1 in]
            n90 = Not Equal?(x=w239, y=w237) -> (x != y?=w238:bool)
            n91 = case shown="True" w238 {
              tunnel: [w247 w248] -> w243
              tunnel: w241 -> [w246 w248]
              tunnel: w240 -> [w245 _]
              tunnel: w237 -> [w244 _]
              frame True {
                n92 = invoke class="VI" method="FP.Open"(reference=w245, error in=w246, "State"=w244) -> (error out=w247:errorcluster)  [unwired: 2 in, 4 out]
              }
              frame False {
              }
            }
          }
        }
        n93 = call <vilib>:"Add State(s) to Queue__JKI_lib_State_Machine.vi"("State(s) in (\"\")"=w188) -> ("States Out"=w187:string)  [unwired: 14 in]
      }
      frame "UI: Update" {
        # "Do not put any code in this frame.\n(It is a separator no-op. You can make a copy of this frame to create a new UI frame)"
        n94 = Unbundle By Name(w256) -> ("Car Wash Data.Car Wash Display.Elapsed Time"=→"Elapsed Time":dbl, "Car Wash Data.Car Wash Display.LED.Under Body Wash"=→"Under Body Wash":bool, "Car Wash Data.Car Wash Display.LED.Bug Remover"=→"Bug Remover":bool, "Car Wash Data.Car Wash Display.LED.Pre-Soak"=→"Pre-Soak":bool, "Car Wash Data.Car Wash Display.LED.High Pressure Wash"=→"High Pressure Wash":bool, "Car Wash Data.Car Wash Display.LED.Low Pressure Wax"=→"Low Pressure Wax":bool, "Car Wash Data.Car Wash Display.LED.Spot Free Rinse"=→"Spot Free Rinse":bool, "Car Wash Data.Car Wash Display.LED.Tire Shine Foam"=→"Tire Shine Foam":bool, "Car Wash Data.Car Wash Display.LED.Air Dry"=→"Air Dry":bool, "Car Wash Data.Car Wash Display.LED.Vehicle out If Position"=→"Vehicle Out Of Position":bool, "Car Wash Data.Car Wash Display.LED.Reading ID"=→"Reading ID":bool, "Car Wash Data.Car Wash Display.LED.Wash Entry"=→"Wash Entry":bool, "Car ID"=→"Current ID":string, "Car Wash Data.Run Mode"=w252:bool)
        n95 = case shown="False" w252 {
          tunnel: w250 -> [w271 _]
          tunnel: [w270 _] -> w251
          frame False {
            w272 = u16 0 items=["Entry", "Station 1", "Station 2", "Station 3", "Exit"] ("Car Position Slider")
            n96 = property on="Car Position Slider" class="Slide (strict)"(error in=w271, "Value"=w272) -> (error out=w270:errorcluster)  [unwired: 1 in, 1 out]
          }
          frame True {
          }
        }
        n97 = Bundle By Name(cluster=w256, "Car Wash Data.Car Position Slider"="Car Position Slider") -> (w257:T9)
        n98 = call <vilib>:"Add State(s) to Queue__JKI_lib_State_Machine.vi"("State(s) in (\"\")"=w269) -> ("States Out"=w268:string)  [unwired: 14 in]
      }
      frame "---------- Macro ----------" {
        # "Do not put any code in this frame.\n(It is a separator no-op. You can make a copy of this frame to create a new Macro frame)"
        n99 = call <vilib>:"Add State(s) to Queue__JKI_lib_State_Machine.vi"("State(s) in (\"\")"=w276) -> ("States Out"=w275:string)  [unwired: 14 in]
      }
      frame "Macro: Initialize" {
        w277 = "Data: Initialize\nInitialize Core Data\nUI: Initialize\nUI: Front Panel State >> Open\nUI: Update\nData: Get DB data\nStatistics: Generate Histogram\nStatistics: The Cleanest Car"  # Data: Initialize Initialize Core Data UI: Initialize UI: Front Panel State >> Open UI: Update Data: Get DB data Statistics: Generate Histogram Statistics: The Cleanest Car
        # "Initialization Macro\n(This is called once, when the VI starts)"
        n100 = call <vilib>:"Add State(s) to Queue__JKI_lib_State_Machine.vi"("State(s) in Front (\"\")"=w277, "State(s) in (\"\")"=w281) -> ("States Out"=w280:string)  [unwired: 13 in]
      }
      frame "Macro: Station 1" {
        # "Exit Macro\n(This is called once, when the VI exits)"
        n101 = call <vilib>:"Add State(s) to Queue__JKI_lib_State_Machine.vi"("State(s) in Front (\"\")"="Action: Under Body Wash\nAction: Bug Remover", "State(s) in (\"\")"=w286) -> ("States Out"=w285:string)  [unwired: 13 in]
      }
      frame "Macro: Station 2" {
        # "Exit Macro\n(This is called once, when the VI exits)"
        n102 = call <vilib>:"Add State(s) to Queue__JKI_lib_State_Machine.vi"("State(s) in Front (\"\")"="Action: Pre Soak\nAction: HP Wash\nAction: LP Wax\nAction: Spot Free Rinse", "State(s) in (\"\")"=w291) -> ("States Out"=w290:string)  [unwired: 13 in]
      }
      frame "Macro: Station 3" {
        # "Exit Macro\n(This is called once, when the VI exits)"
        n103 = call <vilib>:"Add State(s) to Queue__JKI_lib_State_Machine.vi"("State(s) in Front (\"\")"="Action: Tire Shine\nAction: Air Dry", "State(s) in (\"\")"=w296) -> ("States Out"=w295:string)  [unwired: 13 in]
      }
      frame "Macro: Exit" {
        # "Exit Macro\n(This is called once, when the VI exits)"
        n104 = Unbundle By Name(w299) -> ("Core.Close Panel on Exit?"=w298:bool)
        n105 = Select(t="UI: Front Panel State >> Close", s=w298, f="") -> (s? t:f=w301:string)
        n106 = call <vilib>:"Add State(s) to Queue__JKI_lib_State_Machine.vi"("State(s) in (\"\")"=w301, "State(s) at Back (\"\")"="Action: Exit\nUI: Update\nData: Cleanup\nExit") -> ("States Out"=w297:string)  [unwired: 13 in]
        n107 = call <vilib>:"Add State(s) to Queue__JKI_lib_State_Machine.vi"("State(s) in Front (\"\")"=w297, "State(s) in (\"\")"=w306) -> ("States Out"=w305:string)  [unwired: 13 in]
      }
      frame "---------- Action ----------" {
        # "Template Separator\n(You can make a copy of, or modify, this frame)"
        n108 = call <vilib>:"Add State(s) to Queue__JKI_lib_State_Machine.vi"("State(s) in (\"\")"=w310) -> ("States Out"=w309:string)  [unwired: 14 in]
      }
      frame "Action: Start" {
        n109 = call <vilib>:"Add State(s) to Queue__JKI_lib_State_Machine.vi"("State(s) in (\"\")"=w315, "State(s) at Back (\"\")"="Data: Start Configuration\nAction: Set UI Options\nVision: Take photo\nData: DB Insert\nData: Get DB data\nStatistics: Generate Histogram\nStatistics: The Cleanest Car\nMacro: Station 1\nMacro: Station 2\nMacro: Station 3\nAction: Unset UI Options\nUI: Initialize" ("State(s) at Back (\"\")")) -> ("States Out"=w314:string)  [unwired: 13 in]
      }
      frame "Action: Set UI Options" {
        w320 = u16 0 items=["Entry", "Station 1", "Station 2", "Station 3", "Exit"] ("Car Position Slider")
        n110 = property on="Car Position Slider" class="Slide (strict)"(error in=w318, "Value"=w320) -> (error out=w319:errorcluster)  [unwired: 1 in, 1 out]
        n111 = Bundle By Name(cluster=w326, "Car Wash Data.Car Wash Display.LED.Wash Entry"=TRUE, "Car Wash Data.Run Mode"=TRUE, "Car Wash Data.Car Wash Display.LED.Reading ID"=TRUE) -> (w327:T9)
        n112 = property on="Entry Console" class="Clust (strict)"(error in=w319, "DisabledEnum"=T5."Disabled and Grayed Out" ("Disabled")) -> (error out=w323:errorcluster)  [unwired: 1 in, 1 out]
        n113 = property on="Car Position Slider" class="Slide (strict)"(error in=w323, "DisabledEnum"=T5."Enabled" ("Disabled")) -> (error out=w322:errorcluster)  [unwired: 1 in, 1 out]
        n114 = call <vilib>:"Add State(s) to Queue__JKI_lib_State_Machine.vi"("State(s) in (\"\")"=w329) -> ("States Out"=w328:string)  [unwired: 14 in]
      }
      frame "Action: Under Body Wash" {
        n115 = Unbundle By Name(w348) -> ("Car Wash Data.Car Position Slider"=w335:u16, "Car Wash Data.Entry Console.Under Body Wash Button"=w347:bool, "Car Wash Data.Car Wash Display.Reset Stoper"=w333:bool)
        n116 = Select(t=5.0, s=w347, f=0.0) -> (s? t:f=w342:dbl)
        n117 = Equal?(x=w335, y=u16 1 ("Car Wash Data.Car Position Slider")) -> (x = y?=w334:bool)
        n118 = Not(x=w334) -> (.not. x?=w331:bool)
        n119 = call "Timer.vi"("error in (no error)"=w343, "Stop"=w331, "Reset"=w333, "Set time"=w342) -> ("error out"=w344:errorcluster, "Time has Elapsed"=w330:bool, "Time left"=w338:dbl)  [unwired: 5 in]
        n120 = Not Or(1:w331, 2:w330) -> (0:w332:bool)
        n121 = Bundle By Name(cluster=w348, "Car Wash Data.Car Wash Display.Elapsed Time"=w338, "Car Wash Data.Car Wash Display.Reset Stoper"=w330, "Car Wash Data.Car Wash Display.LED.Under Body Wash"=w332, "Car Wash Data.Car Wash Display.LED.Vehicle out If Position"=w331) -> (w349:T9)
        n122 = Select(t="", s=w330, f="Idle\nAction: Under Body Wash") -> (s? t:f=w339:string)
        n123 = call <vilib>:"Add State(s) to Queue__JKI_lib_State_Machine.vi"("State(s) in Front (\"\")"=w339, "State(s) in (\"\")"=w341) -> ("States Out"=w350:string)  [unwired: 13 in]
      }
      frame "Action: Bug Remover" {
        n124 = Unbundle By Name(w369) -> ("Car Wash Data.Car Position Slider"=w356:u16, "Car Wash Data.Entry Console.Bug Remover Button"=w368:bool, "Car Wash Data.Car Wash Display.Reset Stoper"=w354:bool)
        n125 = Select(t=5.0, s=w368, f=0.0) -> (s? t:f=w363:dbl)
        n126 = Equal?(x=w356, y=u16 1 ("Car Wash Data.Car Position Slider")) -> (x = y?=w355:bool)
        n127 = Not(x=w355) -> (.not. x?=w352:bool)
        n128 = call "Timer.vi"("error in (no error)"=w364, "Stop"=w352, "Reset"=w354, "Set time"=w363) -> ("error out"=w365:errorcluster, "Time has Elapsed"=w351:bool, "Time left"=w359:dbl)  [unwired: 5 in]
        n129 = Not Or(1:w352, 2:w351) -> (0:w353:bool)
        n130 = Bundle By Name(cluster=w369, "Car Wash Data.Car Wash Display.Elapsed Time"=w359, "Car Wash Data.Car Wash Display.Reset Stoper"=w351, "Car Wash Data.Car Wash Display.LED.Bug Remover"=w353, "Car Wash Data.Car Wash Display.LED.Vehicle out If Position"=w352) -> (w370:T9)
        n131 = Select(t="", s=w351, f="Idle\nAction: Bug Remover") -> (s? t:f=w360:string)
        n132 = call <vilib>:"Add State(s) to Queue__JKI_lib_State_Machine.vi"("State(s) in Front (\"\")"=w360, "State(s) in (\"\")"=w362) -> ("States Out"=w371:string)  [unwired: 13 in]
      }
      frame "Action: Pre Soak" {
        n133 = Unbundle By Name(w390) -> ("Car Wash Data.Car Position Slider"=w377:u16, "Car Wash Data.Entry Console.Pre-Soak Button"=w389:bool, "Car Wash Data.Car Wash Display.Reset Stoper"=w375:bool)
        n134 = Select(t=5.0, s=w389, f=0.0) -> (s? t:f=w384:dbl)
        n135 = Equal?(x=w377, y=u16 2 ("Car Wash Data.Car Position Slider")) -> (x = y?=w376:bool)
        n136 = Not(x=w376) -> (.not. x?=w373:bool)
        n137 = call "Timer.vi"("error in (no error)"=w385, "Stop"=w373, "Reset"=w375, "Set time"=w384) -> ("error out"=w386:errorcluster, "Time has Elapsed"=w372:bool, "Time left"=w380:dbl)  [unwired: 5 in]
        n138 = Not Or(1:w373, 2:w372) -> (0:w374:bool)
        n139 = Bundle By Name(cluster=w390, "Car Wash Data.Car Wash Display.Elapsed Time"=w380, "Car Wash Data.Car Wash Display.Reset Stoper"=w372, "Car Wash Data.Car Wash Display.LED.Pre-Soak"=w374, "Car Wash Data.Car Wash Display.LED.Vehicle out If Position"=w373) -> (w391:T9)
        n140 = Select(t="", s=w372, f="Idle\nAction: Pre Soak") -> (s? t:f=w381:string)
        n141 = call <vilib>:"Add State(s) to Queue__JKI_lib_State_Machine.vi"("State(s) in Front (\"\")"=w381, "State(s) in (\"\")"=w383) -> ("States Out"=w392:string)  [unwired: 13 in]
      }
      frame "Action: HP Wash" {
        n142 = Unbundle By Name(w411) -> ("Car Wash Data.Car Position Slider"=w398:u16, "Car Wash Data.Entry Console.High Pressure Wash Button"=w410:bool, "Car Wash Data.Car Wash Display.Reset Stoper"=w396:bool)
        n143 = Select(t=5.0, s=w410, f=0.0) -> (s? t:f=w405:dbl)
        n144 = Equal?(x=w398, y=u16 2 ("Car Wash Data.Car Position Slider")) -> (x = y?=w397:bool)
        n145 = Not(x=w397) -> (.not. x?=w394:bool)
        n146 = call "Timer.vi"("error in (no error)"=w406, "Stop"=w394, "Reset"=w396, "Set time"=w405) -> ("error out"=w407:errorcluster, "Time has Elapsed"=w393:bool, "Time left"=w401:dbl)  [unwired: 5 in]
        n147 = Not Or(1:w394, 2:w393) -> (0:w395:bool)
        n148 = Bundle By Name(cluster=w411, "Car Wash Data.Car Wash Display.Elapsed Time"=w401, "Car Wash Data.Car Wash Display.Reset Stoper"=w393, "Car Wash Data.Car Wash Display.LED.High Pressure Wash"=w395, "Car Wash Data.Car Wash Display.LED.Vehicle out If Position"=w394) -> (w412:T9)
        n149 = Select(t="", s=w393, f="Idle\nAction: HP Wash") -> (s? t:f=w402:string)
        n150 = call <vilib>:"Add State(s) to Queue__JKI_lib_State_Machine.vi"("State(s) in Front (\"\")"=w402, "State(s) in (\"\")"=w404) -> ("States Out"=w413:string)  [unwired: 13 in]
      }
      frame "Action: LP Wax" {
        n151 = Unbundle By Name(w432) -> ("Car Wash Data.Car Position Slider"=w419:u16, "Car Wash Data.Entry Console.Low Pressure Wax Button"=w431:bool, "Car Wash Data.Car Wash Display.Reset Stoper"=w417:bool)
        n152 = Select(t=5.0, s=w431, f=0.0) -> (s? t:f=w426:dbl)
        n153 = Equal?(x=w419, y=u16 2 ("Car Wash Data.Car Position Slider")) -> (x = y?=w418:bool)
        n154 = Not(x=w418) -> (.not. x?=w415:bool)
        n155 = call "Timer.vi"("error in (no error)"=w427, "Stop"=w415, "Reset"=w417, "Set time"=w426) -> ("error out"=w428:errorcluster, "Time has Elapsed"=w414:bool, "Time left"=w422:dbl)  [unwired: 5 in]
        n156 = Not Or(1:w415, 2:w414) -> (0:w416:bool)
        n157 = Bundle By Name(cluster=w432, "Car Wash Data.Car Wash Display.Elapsed Time"=w422, "Car Wash Data.Car Wash Display.Reset Stoper"=w414, "Car Wash Data.Car Wash Display.LED.Low Pressure Wax"=w416, "Car Wash Data.Car Wash Display.LED.Vehicle out If Position"=w415) -> (w433:T9)
        n158 = Select(t="", s=w414, f="Idle\nAction: LP Wax") -> (s? t:f=w423:string)
        n159 = call <vilib>:"Add State(s) to Queue__JKI_lib_State_Machine.vi"("State(s) in Front (\"\")"=w423, "State(s) in (\"\")"=w425) -> ("States Out"=w434:string)  [unwired: 13 in]
      }
      frame "Action: Spot Free Rinse" {
        n160 = Unbundle By Name(w453) -> ("Car Wash Data.Car Position Slider"=w440:u16, "Car Wash Data.Entry Console.Spot Free Rinse Button"=w452:bool, "Car Wash Data.Car Wash Display.Reset Stoper"=w438:bool)
        n161 = Select(t=5.0, s=w452, f=0.0) -> (s? t:f=w447:dbl)
        n162 = Equal?(x=w440, y=u16 2 ("Car Wash Data.Car Position Slider")) -> (x = y?=w439:bool)
        n163 = Not(x=w439) -> (.not. x?=w436:bool)
        n164 = call "Timer.vi"("error in (no error)"=w448, "Stop"=w436, "Reset"=w438, "Set time"=w447) -> ("error out"=w449:errorcluster, "Time has Elapsed"=w435:bool, "Time left"=w443:dbl)  [unwired: 5 in]
        n165 = Not Or(1:w436, 2:w435) -> (0:w437:bool)
        n166 = Bundle By Name(cluster=w453, "Car Wash Data.Car Wash Display.Elapsed Time"=w443, "Car Wash Data.Car Wash Display.Reset Stoper"=w435, "Car Wash Data.Car Wash Display.LED.Spot Free Rinse"=w437, "Car Wash Data.Car Wash Display.LED.Vehicle out If Position"=w436) -> (w454:T9)
        n167 = Select(t="", s=w435, f="Idle\nAction: Spot Free Rinse") -> (s? t:f=w444:string)
        n168 = call <vilib>:"Add State(s) to Queue__JKI_lib_State_Machine.vi"("State(s) in Front (\"\")"=w444, "State(s) in (\"\")"=w446) -> ("States Out"=w455:string)  [unwired: 13 in]
      }
      frame "Action: Tire Shine" {
        n169 = Unbundle By Name(w474) -> ("Car Wash Data.Car Position Slider"=w461:u16, "Car Wash Data.Entry Console.Tire Shine Foam Button"=w473:bool, "Car Wash Data.Car Wash Display.Reset Stoper"=w459:bool)
        n170 = Select(t=5.0, s=w473, f=0.0) -> (s? t:f=w468:dbl)
        n171 = Equal?(x=w461, y=u16 3 ("Car Wash Data.Car Position Slider")) -> (x = y?=w460:bool)
        n172 = Not(x=w460) -> (.not. x?=w457:bool)
        n173 = call "Timer.vi"("error in (no error)"=w469, "Stop"=w457, "Reset"=w459, "Set time"=w468) -> ("error out"=w470:errorcluster, "Time has Elapsed"=w456:bool, "Time left"=w464:dbl)  [unwired: 5 in]
        n174 = Not Or(1:w457, 2:w456) -> (0:w458:bool)
        n175 = Bundle By Name(cluster=w474, "Car Wash Data.Car Wash Display.Elapsed Time"=w464, "Car Wash Data.Car Wash Display.Reset Stoper"=w456, "Car Wash Data.Car Wash Display.LED.Tire Shine Foam"=w458, "Car Wash Data.Car Wash Display.LED.Vehicle out If Position"=w457) -> (w475:T9)
        n176 = Select(t="", s=w456, f="Idle\nAction: Tire Shine ") -> (s? t:f=w465:string)
        n177 = call <vilib>:"Add State(s) to Queue__JKI_lib_State_Machine.vi"("State(s) in Front (\"\")"=w465, "State(s) in (\"\")"=w467) -> ("States Out"=w476:string)  [unwired: 13 in]
      }
      frame "Action: Air Dry" {
        n178 = Unbundle By Name(w495) -> ("Car Wash Data.Car Position Slider"=w482:u16, "Car Wash Data.Entry Console.Air Dry"=w494:bool, "Car Wash Data.Car Wash Display.Reset Stoper"=w480:bool)
        n179 = Select(t=5.0, s=w494, f=0.0) -> (s? t:f=w489:dbl)
        n180 = Equal?(x=w482, y=u16 3 ("Car Wash Data.Car Position Slider")) -> (x = y?=w481:bool)
        n181 = Not(x=w481) -> (.not. x?=w478:bool)
        n182 = call "Timer.vi"("error in (no error)"=w490, "Stop"=w478, "Reset"=w480, "Set time"=w489) -> ("error out"=w491:errorcluster, "Time has Elapsed"=w477:bool, "Time left"=w485:dbl)  [unwired: 5 in]
        n183 = Not Or(1:w478, 2:w477) -> (0:w479:bool)
        n184 = Bundle By Name(cluster=w495, "Car Wash Data.Car Wash Display.Elapsed Time"=w485, "Car Wash Data.Car Wash Display.Reset Stoper"=w477, "Car Wash Data.Car Wash Display.LED.Air Dry"=w479, "Car Wash Data.Car Wash Display.LED.Vehicle out If Position"=w478) -> (w496:T9)
        n185 = Select(t="", s=w477, f="Idle\nAction: Air Dry") -> (s? t:f=w486:string)
        n186 = call <vilib>:"Add State(s) to Queue__JKI_lib_State_Machine.vi"("State(s) in Front (\"\")"=w486, "State(s) in (\"\")"=w488) -> ("States Out"=w497:string)  [unwired: 13 in]
      }
      frame "Action: Unset UI Options" {
        n187 = Unbundle By Name(w503) -> ("Car Wash Data.Car Position Slider"=w508:u16)
        n188 = Equal?(x=w508, y=u16 4) -> (x = y?=w504:bool)
        n189 = case shown="True" w504 {
          selector: w504 -> [w511 w526]
          tunnel: w506 -> [w513 w521]
          tunnel: [w513 w520] -> w505
          tunnel: w503 -> [w512 w528]
          tunnel: [w512 w527] -> w502
          tunnel: [w511 w526] -> w500
          frame False {
          }
          frame True {
            w518 = u16 0 items=["Entry", "Station 1", "Station 2", "Station 3", "Exit"] ("Car Position Slider")
            n190 = property on="Entry Console" class="Clust (strict)"(error in=w521, "DisabledEnum"=T5."Enabled" ("Disabled")) -> (error out=w523:errorcluster)  [unwired: 1 in, 1 out]
            n191 = Bundle By Name(cluster=w528, "Car Wash Data.Car Wash Display.LED"=T7 {"Under Body Wash"=FALSE, "Bug Remover"=FALSE, "Pre-Soak"=FALSE, "High Pressure Wash"=FALSE, "Low Pressure Wax"=FALSE, "Spot Free Rinse"=FALSE, "Tire Shine Foam"=FALSE, "Air Dry"=FALSE, "Vehicle out If Position"=FALSE, "Wash Entry"=FALSE, "Reading ID"=FALSE}, "Car Wash Data.Run Mode"=FALSE, "Car Wash Data.Car Wash Display.LED.Reading ID"=FALSE) -> (w527:T9)
            n192 = property on="Entry Console" class="Clust (strict)"(error in=w523, "Value"=T6 {"Under Body Wash Button"=FALSE, "Bug Remover Button"=FALSE, "Pre-Soak Button"=FALSE, "High Pressure Wash Button"=FALSE, "Low Pressure Wax Button"=FALSE, "Spot Free Rinse Button"=FALSE, "Tire Shine Foam Button"=FALSE, "Air Dry"=FALSE} ("Entry Console")) -> (error out=w517:errorcluster)  [unwired: 1 in, 1 out]
            n193 = property on="Car Position Slider" class="Slide (strict)"(error in=w517, "Value"=w518) -> (error out=w516:errorcluster)  [unwired: 1 in, 1 out]
            n194 = property on="Car Position Slider" class="Slide (strict)"(error in=w516, "DisabledEnum"=T5."Disabled" ("Disabled")) -> (error out=w520:errorcluster)  [unwired: 1 in, 1 out]
          }
        }
        n195 = Select(t="", s=w500, f="Idle\nAction: Unset UI Options") -> (s? t:f=w499:string)
        n196 = call <vilib>:"Add State(s) to Queue__JKI_lib_State_Machine.vi"("State(s) in Front (\"\")"=w499, "State(s) in (\"\")"=w510) -> ("States Out"=w509:string)  [unwired: 13 in]
      }
      frame "Action: Exit" {
        w539 = u16 0 items=["Entry", "Station 1", "Station 2", "Station 3", "Exit"] ("Car Position Slider")
        n197 = property on="Entry Console" class="Clust (strict)"(error in=w530, "DisabledEnum"=T5."Enabled" ("Disabled")) -> (error out=w531:errorcluster)  [unwired: 1 in, 1 out]
        n198 = property on="Entry Console" class="Clust (strict)"(error in=w531, "Value"=T6 {"Under Body Wash Button"=FALSE, "Bug Remover Button"=FALSE, "Pre-Soak Button"=FALSE, "High Pressure Wash Button"=FALSE, "Low Pressure Wax Button"=FALSE, "Spot Free Rinse Button"=FALSE, "Tire Shine Foam Button"=FALSE, "Air Dry"=FALSE} ("Entry Console")) -> (error out=w533:errorcluster)  [unwired: 1 in, 1 out]
        n199 = Bundle By Name(cluster=w535, "Car Wash Data.Car Wash Display.Elapsed Time"=0.0, "Car Wash Data.Car Wash Display.LED"=T7 {"Under Body Wash"=FALSE, "Bug Remover"=FALSE, "Pre-Soak"=FALSE, "High Pressure Wash"=FALSE, "Low Pressure Wax"=FALSE, "Spot Free Rinse"=FALSE, "Tire Shine Foam"=FALSE, "Air Dry"=FALSE, "Vehicle out If Position"=FALSE, "Wash Entry"=FALSE, "Reading ID"=FALSE} ("Car Wash Display.LED")) -> (w536:T9)
        n200 = property on="Car Position Slider" class="Slide (strict)"(error in=w533, "Value"=w539) -> (error out=w538:errorcluster)  [unwired: 1 in, 1 out]
        n201 = call <vilib>:"Add State(s) to Queue__JKI_lib_State_Machine.vi"("State(s) in (\"\")"=w541) -> ("States Out"=w540:string)  [unwired: 14 in]
      }
      frame "---------- Statistics ----------" {
        # "Template Separator\n(You can make a copy of, or modify, this frame)"
        n202 = call <vilib>:"Add State(s) to Queue__JKI_lib_State_Machine.vi"("State(s) in (\"\")"=w545) -> ("States Out"=w544:string)  [unwired: 14 in]
      }
      frame "Statistics: Generate Histogram" {
        w547 = i32[] [1, 2, 3, 4, 5, 6, 7, 8]  # Options (1-8)
        # "Template Separator\n(You can make a copy of, or modify, this frame)"
        n203 = Unbundle By Name(w552) -> ("SQLite Connection"=w549:refnum<class "Connection.lvclass">)
        n204 = call "DB_SelectSum.vi"("error in (no error)"=w550, "SQLite Connection in"=w549) -> ("error out"=w551:errorcluster, "Array"=w546:i64[])  [unwired: 7 in, 1 out]
        n205 = Bundle("Options (1-8)"=w547, "Array"=w546) -> (→"Histogram":cluster{"Options (1-8)":i32[], "Array":i64[]})  [unwired: 1 in]
        n206 = call <vilib>:"Add State(s) to Queue__JKI_lib_State_Machine.vi"("State(s) in (\"\")"=w554) -> ("States Out"=w553:string)  [unwired: 14 in]
      }
      frame "Statistics: The Cleanest Car" {
        # "Template Separator\n(You can make a copy of, or modify, this frame)"
        n207 = Unbundle By Name(w559) -> ("SQLite Connection"=w556:refnum<class "Connection.lvclass">)
        n208 = call "DB_GetMostFrequentID.vi"("error in (no error)"=w558, "SQLite Connection in"=w556) -> ("error out"=w557:errorcluster, "Most Frequent ID"=→"Cleanest Car ID":string[])  [unwired: 8 in]
        n209 = call <vilib>:"Add State(s) to Queue__JKI_lib_State_Machine.vi"("State(s) in (\"\")"=w561) -> ("States Out"=w560:string)  [unwired: 14 in]
      }
      frame "---------- Vision----------" {
        # "Template Separator\n(You can make a copy of, or modify, this frame)"
        n210 = call <vilib>:"Add State(s) to Queue__JKI_lib_State_Machine.vi"("State(s) in (\"\")"=w565) -> ("States Out"=w564:string)  [unwired: 14 in]
      }
      frame "Vision: Take photo" {
        n211 = call "Take_photo.vi"("error in"=w567, "Session In"="Choose camera") -> ("error out"=w568:errorcluster, "x = y?"=w566:bool)  [unwired: 7 in]
        n212 = Select(t="Vision: OCR", s=w566, f="Idle\nVision: Take photo") -> (s? t:f=w572:string)
        n213 = call <vilib>:"Add State(s) to Queue__JKI_lib_State_Machine.vi"("State(s) in Front (\"\")"=w572, "State(s) in (\"\")"=w575) -> ("States Out"=w574:string)  [unwired: 13 in]
      }
      frame "Vision: OCR" {
        n214 = call "OCR.vi"("error in (no error)"=w582) -> ("error out"=w581:errorcluster, "Read String"=w580:string)  [unwired: 9 in]
        n215 = Bundle By Name(cluster=w578, "Car ID"=w580, "Car Wash Data.Car Wash Display.LED.Reading ID"=FALSE) -> (w579:T9)
        n216 = call <vilib>:"Add State(s) to Queue__JKI_lib_State_Machine.vi"("State(s) in Front (\"\")"="", "State(s) in (\"\")"=w584) -> ("States Out"=w583:string)  [unwired: 13 in]
      }
    }
  }
